vi "Transmit.vi"(8 "error in (no error)":errorcluster, 9 "timeout in ms (-1)":i32=-1, 10 "Packet":refnum<class "Packet.lvclass">, 11 "Communication In":refnum<class "IP_Communication.lvclass">) -> (0 "error out":errorcluster, 1 "Timeout?":bool, 2 "Packet Sent":refnum<class "Packet.lvclass">, 3 "Communication Out":refnum<class "IP_Communication.lvclass">)   [LabVIEW 2020, in "Communication Classes.lvlib" / "IP_Communication.lvclass"]
uses:
  IP_Communication.lvclass
  Packet/Packet.lvclass
  IP_Communication.lvclass/IP_Communication.ctl
  Packet/Packet.lvclass/Packet.ctl
  <vilib>/Utility/error.llb/Error Cluster From Error Code.vi
  <vilib>/ErrorRing/Error Ring.xnode
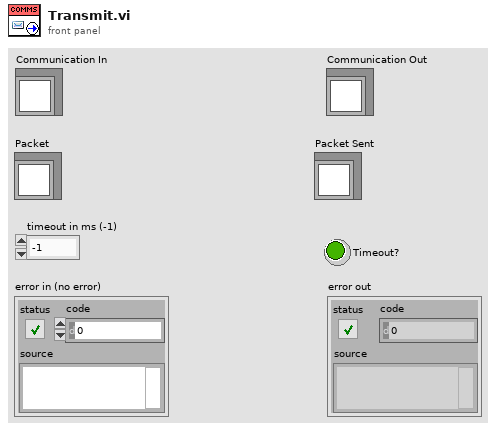
[diagram p1: front panel]
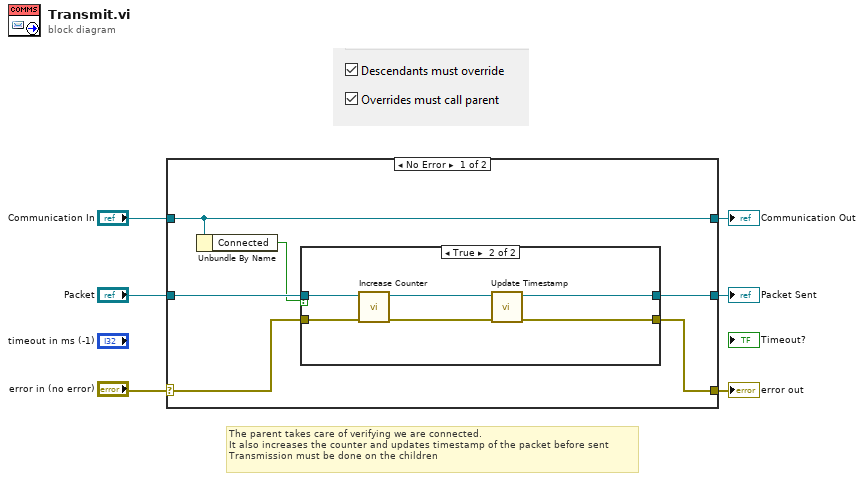
[diagram p0: block diagram]
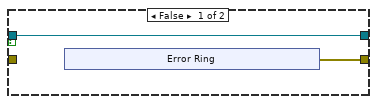
[diagram p2: hidden frame]
diagram:
  # "The parent takes care of verifying we are connected.\nIt also increases the counter and updates timestamp of the packet before sent\nTransmission must be done on the children"
  n1 = case shown="No Error" "error in (no error)" {
    selector: "error in (no error)" -> [w11 w27]
    tunnel: "Communication In" -> [w8 w28]
    tunnel: [w8 w28] -> w5
    tunnel: [w9 w27] -> w3
    tunnel: "Packet" -> [w12 w26]
    tunnel: [w10 w26] -> w1
    frame No Error {
      n2 = Unbundle By Name(w8) -> ("Connected"=w7:bool)
      n3 = case shown="True" w7 {
        tunnel: w12 -> [w14 w25]
        tunnel: w11 -> [_ w22]
        tunnel: [w14 w21] -> w10
        tunnel: [w13 w20] -> w9
        frame False {
          n4 = xnode "Error Ring"() -> ("error out"=w13:errorcluster)
        }
        frame True {
          n5 = call "Increase Counter.vi"("error in (no error)"=w22, "Packet in"=w25) -> ("error out"=w23:errorcluster, "Packet out"=w24:refnum<class "Packet.lvclass">)  [unwired: 8 in]
          n6 = call "Update Timestamp.vi"("error in (no error)"=w23, "Packet in"=w24) -> ("error out"=w20:errorcluster, "Packet out"=w21:refnum<class "Packet.lvclass">)  [unwired: 8 in]
        }
      }
    }
    frame Error {
    }
  }
  "Communication Out" <- w5
  "error out" <- w3
  "Packet Sent" <- w1
